vi "Adder.vi"() -> ()   [LabVIEW 2012]
uses:
  SimpleAdder/SimpleAdder.lvclass
  messagelib/TAS_Message.lvclass
  SimpleAdder/SimpleAdder.lvclass/SimpleAdder.ctl
  SimpleAdder/Message/AdderMsg.lvclass
panel:
  out "Sum":dbl
  in  "Process Stop Button":bool
  in  "Add!":bool
  in  "Addend 2":dbl
  in  "Addend 1":dbl
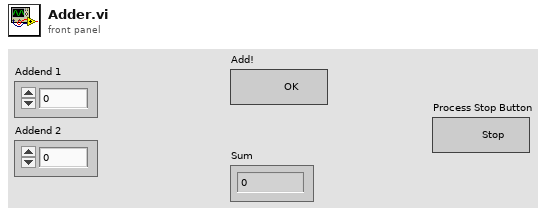
[diagram p1: front panel]
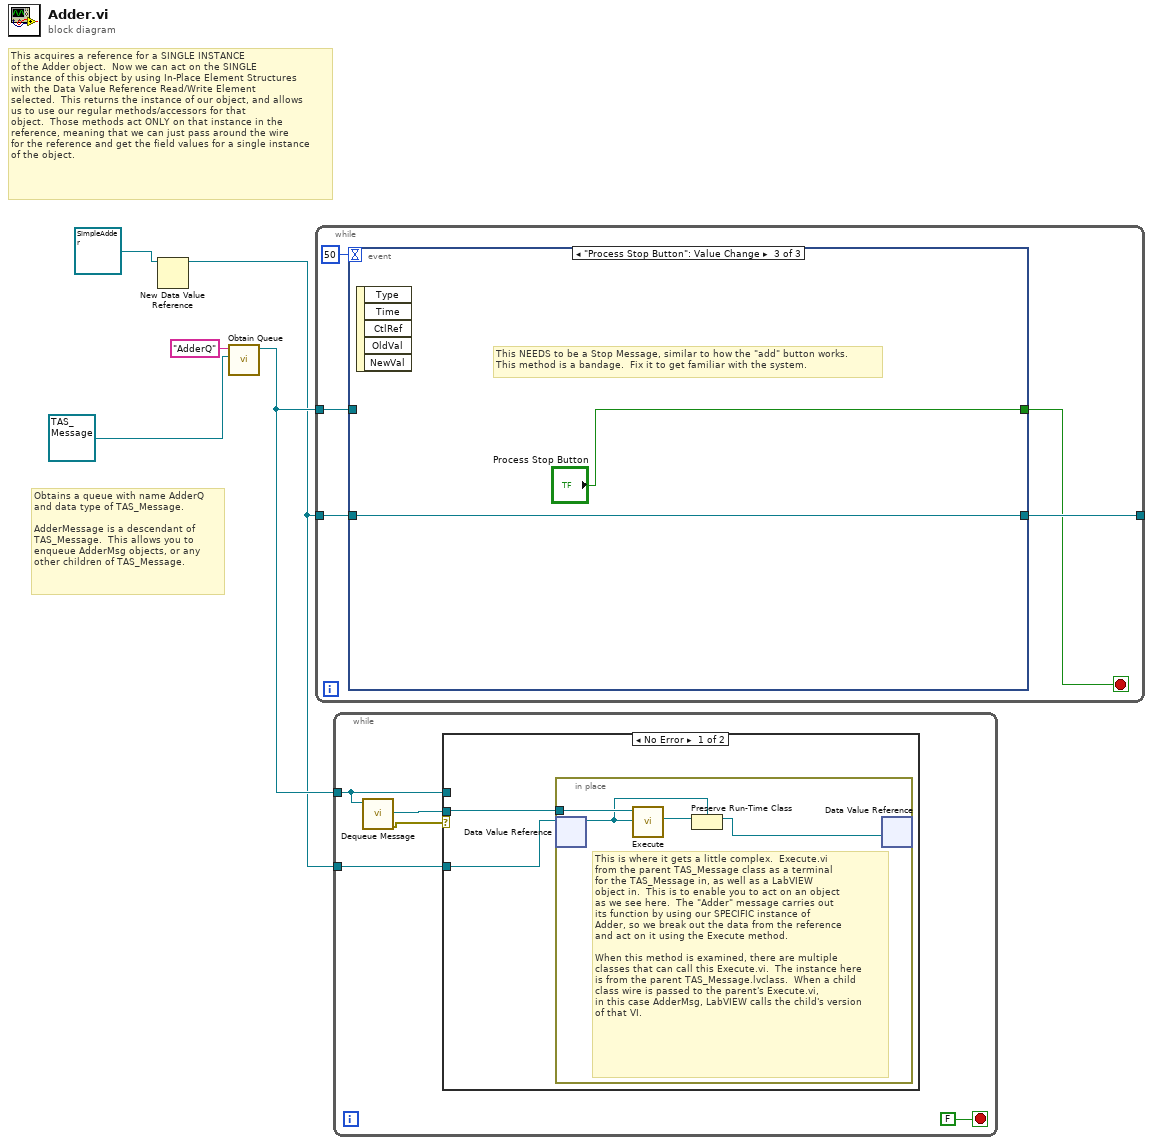
[diagram p0: block diagram]
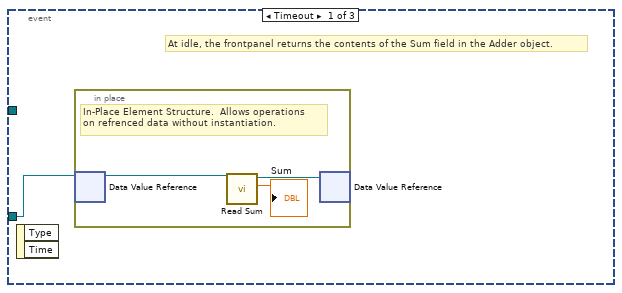
[diagram p3: hidden frame]
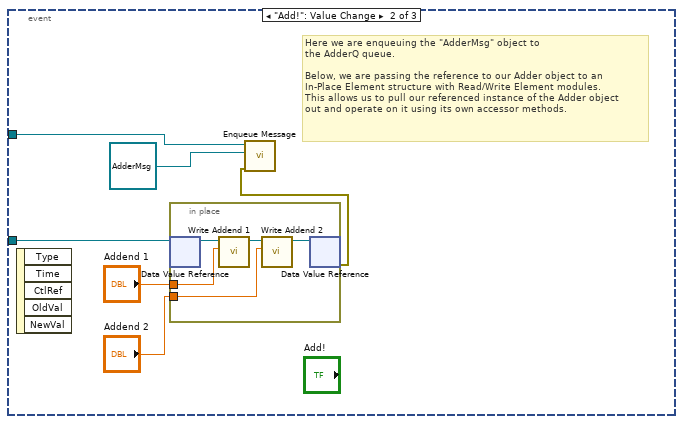
[diagram p4: hidden frame]
diagram:
  # "Obtains a queue with name AdderQ\nand data type of TAS_Message.\n\nAdderMessage is a descendant of \nTAS_Message.  This allows you to \nenqueue AdderMsg objects, or any\nother children of TAS_Message."
  # "This acquires a reference for a SINGLE INSTANCE\nof the Adder object.  Now we can act on the SINGLE \ninstance of this object by using In-Place Element Structures\nwith the Data Value Reference Read/Write Element\nselected.  This returns the instance of our object, and allows\nus to use our regular methods/accessors for that\nobject.  Those methods act ONLY on that instance in the \nreference, meaning that we can just pass around the wire\nfor the reference and get the field values for a single instance\nof the object."
  n1 = New Data Value Reference(data value=refnum<class "SimpleAdder.lvclass"> refnum ("SimpleAdder.lvclass")) -> (data value reference=w2:refnum<data-value>)  [unwired: 1 in, 1 out]
  n2 = call-dynamic "Obtain Queue.vi"("TAS_Message.lvclass"=refnum<class "TAS_Message.lvclass"> refnum, "Queue Name"="AdderQ") -> ("queue out"=w4:refnum<queue>)  [unwired: 8 in, 1 out]
  n3 = while {
    tunnel: w4 -> [w10]
    tunnel: w2 -> [w9]
    tunnel: [w7] -> _
    stop <- w6 stop-if-true
    n4 = event shown="[2] \"Process Stop Button\": Value Change" {
      selector: _ -> [_ _ _]
      dyn-events: _ -> [_ _ _]
      timeout: 50 -> [_ _ _]
      tunnel: w10 -> [_ w19 _]
      tunnel: w9 -> [w11 w18 w26]
      tunnel: [_ _ "Process Stop Button"] -> w6
      tunnel: [_ _ w26] -> w7
      event Timeout {
        # "At idle, the frontpanel returns the contents of the Sum field in the Adder object."
        n5 = event-data() -> ()  [unwired: 1 in, 2 out]
        n6 = in-place {
          # "In-Place Element Structure.  Allows operations\non refrenced data without instantiation."
          n7 = in-place-dvr #1(w11) -> (w13:refnum<class "SimpleAdder.lvclass">)  [unwired: 1 out]
          n8 = call "Read Sum.vi"("SimpleAdder in"=w13) -> ("Sum"=→"Sum":dbl, "SimpleAdder out"=w12:refnum<class "SimpleAdder.lvclass">)  [unwired: 8 in, 1 out]
          n9 = in-place-dvr #1(w12) -> ()  [unwired: 2 out]
        }
      }
      event "Add!": Value Change {
        # "Here we are enqueuing the \"AdderMsg\" object to\nthe AdderQ queue.\n\nBelow, we are passing the reference to our Adder object to an\nIn-Place Element structure with Read/Write Element modules.\nThis allows us to pull our referenced instance of the Adder object\nout and operate on it using its own accessor methods."
        n10 = event-data() -> ()  [unwired: 1 in, 5 out]
        n11 = in-place {
          in-place-border: "Addend 2" -> [w24]
          in-place-border: "Addend 1" -> [w23]
          n12 = in-place-dvr #2(w18) -> (w25:refnum<class "SimpleAdder.lvclass">)  [unwired: 1 out]
          n13 = call "Write Addend 1.vi"("Addend 1"=w23, "SimpleAdder in"=w25) -> ("SimpleAdder out"=w22:refnum<class "SimpleAdder.lvclass">)  [unwired: 8 in, 1 out]
          n14 = call "Write Addend 2.vi"("Addend 2"=w24, "SimpleAdder in"=w22) -> ("SimpleAdder out"=w21:refnum<class "SimpleAdder.lvclass">)  [unwired: 8 in, 1 out]
          n15 = in-place-dvr #2(w21) -> (w15:errorcluster)  [unwired: 1 out]
        }
        n16 = call-dynamic "Enqueue Message.vi"("error in (no error)"=w15, "Queue Element In"=refnum<class "AdderMsg.lvclass"> refnum ("AdderMsg.lvclass"), "TAS_Message queue in"=w19) -> ()  [unwired: 7 in, 2 out]
      }
      event "Process Stop Button": Value Change {
        # "This NEEDS to be a Stop Message, similar to how the \"add\" button works.\nThis method is a bandage.  Fix it to get familiar with the system."
        n17 = event-data() -> ()  [unwired: 1 in, 5 out]
      }
    }
  }
  n18 = while {
    tunnel: w4 -> [w32]
    tunnel: w2 -> [w29]
    stop <- FALSE stop-if-true
    n19 = call "Dequeue Message.vi"("TAS_Message queue in"=w32) -> ("error out"=w31:errorcluster, "Queue Element Out"=w30:refnum<class "TAS_Message.lvclass">)  [unwired: 8 in, 1 out]
    n20 = case shown="No Error" w31 {
      tunnel: w32 -> [_ _]
      tunnel: w30 -> [w33 _]
      tunnel: w29 -> [w34 _]
      frame No Error {
        n21 = in-place {
          in-place-border: w33 -> [w38]
          # "This is where it gets a little complex.  Execute.vi\nfrom the parent TAS_Message class as a terminal\nfor the TAS_Message in, as well as a LabVIEW\nobject in.  This is to enable you to act on an object\nas we see here.  The \"Adder\" message carries out\nits function by using our SPECIFIC instance of\nAdder, so we break out the data from the reference\nand act on it using the Execute method.\n\nWhen this method is examined, there are multiple\nclasses that can call this Execute.vi.  The instance here\nis from the parent TAS_Message.lvclass.  When a child\nclass wire is passed to the parent's Execute.vi,\nin this case AdderMsg, LabVIEW calls the child's version\nof that VI."
          n22 = in-place-dvr #3(w34) -> (w36:refnum<class "SimpleAdder.lvclass">)  [unwired: 1 out]
          n23 = call-dynamic "Execute.vi"("LabVIEW Object In"=w36, "TAS_Message in"=w38) -> ("LabVIEW Object Out"=w37:refnum<class>)  [unwired: 7 in, 2 out]
          n24 = Preserve Run-Time Class(object in=w37, 2:w36) -> (object out=w35:refnum<class "SimpleAdder.lvclass">)  [unwired: 1 in, 1 out]
          n25 = in-place-dvr #3(w35) -> ()  [unwired: 2 out]
        }
      }
      frame Error {
      }
    }
  }
